vi "mainhex.vi"() -> ()   [LabVIEW 2018]
uses:
  <vilib>/Instr/_visa.llb/VISA Configure Serial Port (Instr).vi
panel:
  out "Log file path":path
  in  "Project Name":string="BDC_prototype"
  out "Bat current":dbl caption="Current Temperature\n(Celsius)"
  out "Bat current":cluster{dbl[], dbl[]}(graph)
  out "Bat Voltage":dbl caption="Current Temperature\n(Celsius)"
  out "Bat voltage":cluster{dbl[], dbl[]}(graph)
  out "Time":dbl caption="Current Temperature\n(Celsius)"
  out "String":string
  in  "stop":bool
  out "Bus Voltage":dbl caption="Current Temperature\n(Celsius)"
  out "Bus voltage":cluster{dbl[], dbl[]}(graph)
  in  "Port":refnum<visa-resource-name>="COM5"
  in  "Baud rate":u32=57600
  in  "Data bits (8)":u16=8 min=5 max=8 step=1
  in  "Stop bits (1)":u16(ring)=10 items=["1.0"=10, "1.5"=15, "2.0"=20]
  in  "Flow control (None)":u16(ring) items=["None", "XON/XOFF", "RTS/CTS", "XON/XOFF & RTS/CTS", "DTR/DSR", "XON/XOFF & DTR/DSR"]
  in  "Parity (None)":enum16{"None", "Odd", "Even", "Mark", "Space"}(ring)
  # "UART"
  # "FILES"
  # "ACTIONS"
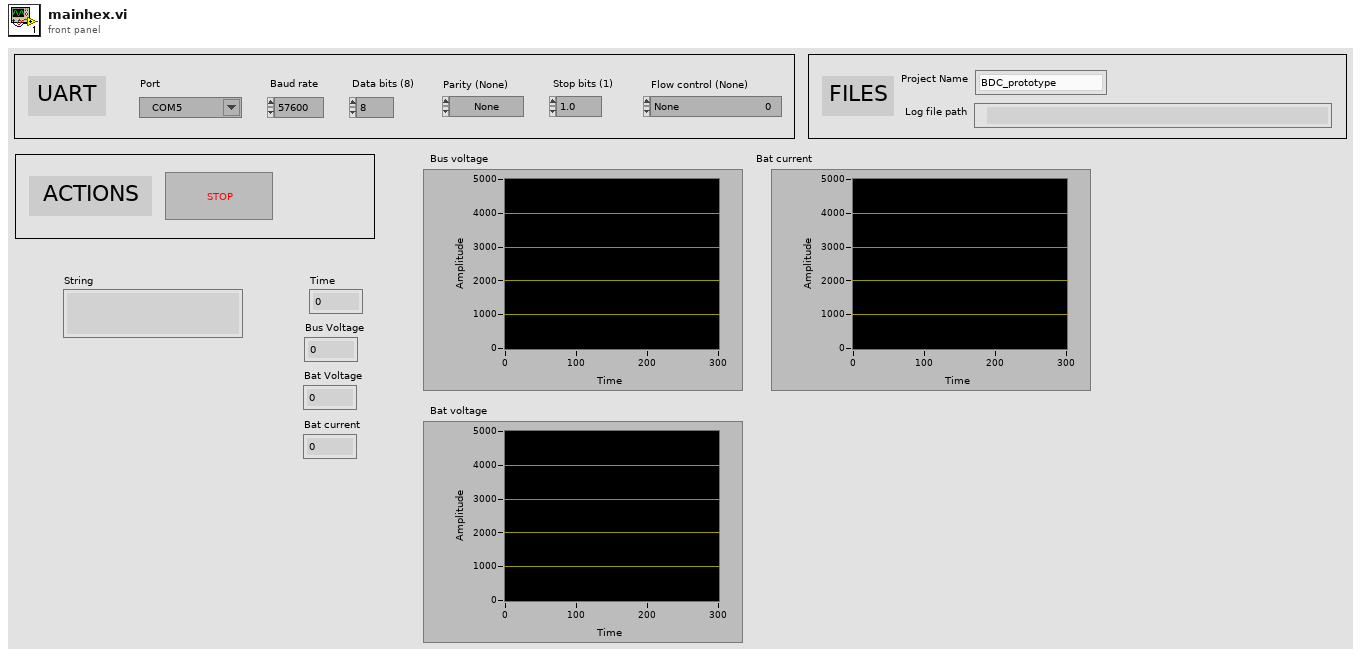
[diagram p1: front panel]
types:
  T1 = enum16{"open", "open or create", "create or replace", "create", "open (read only)"}
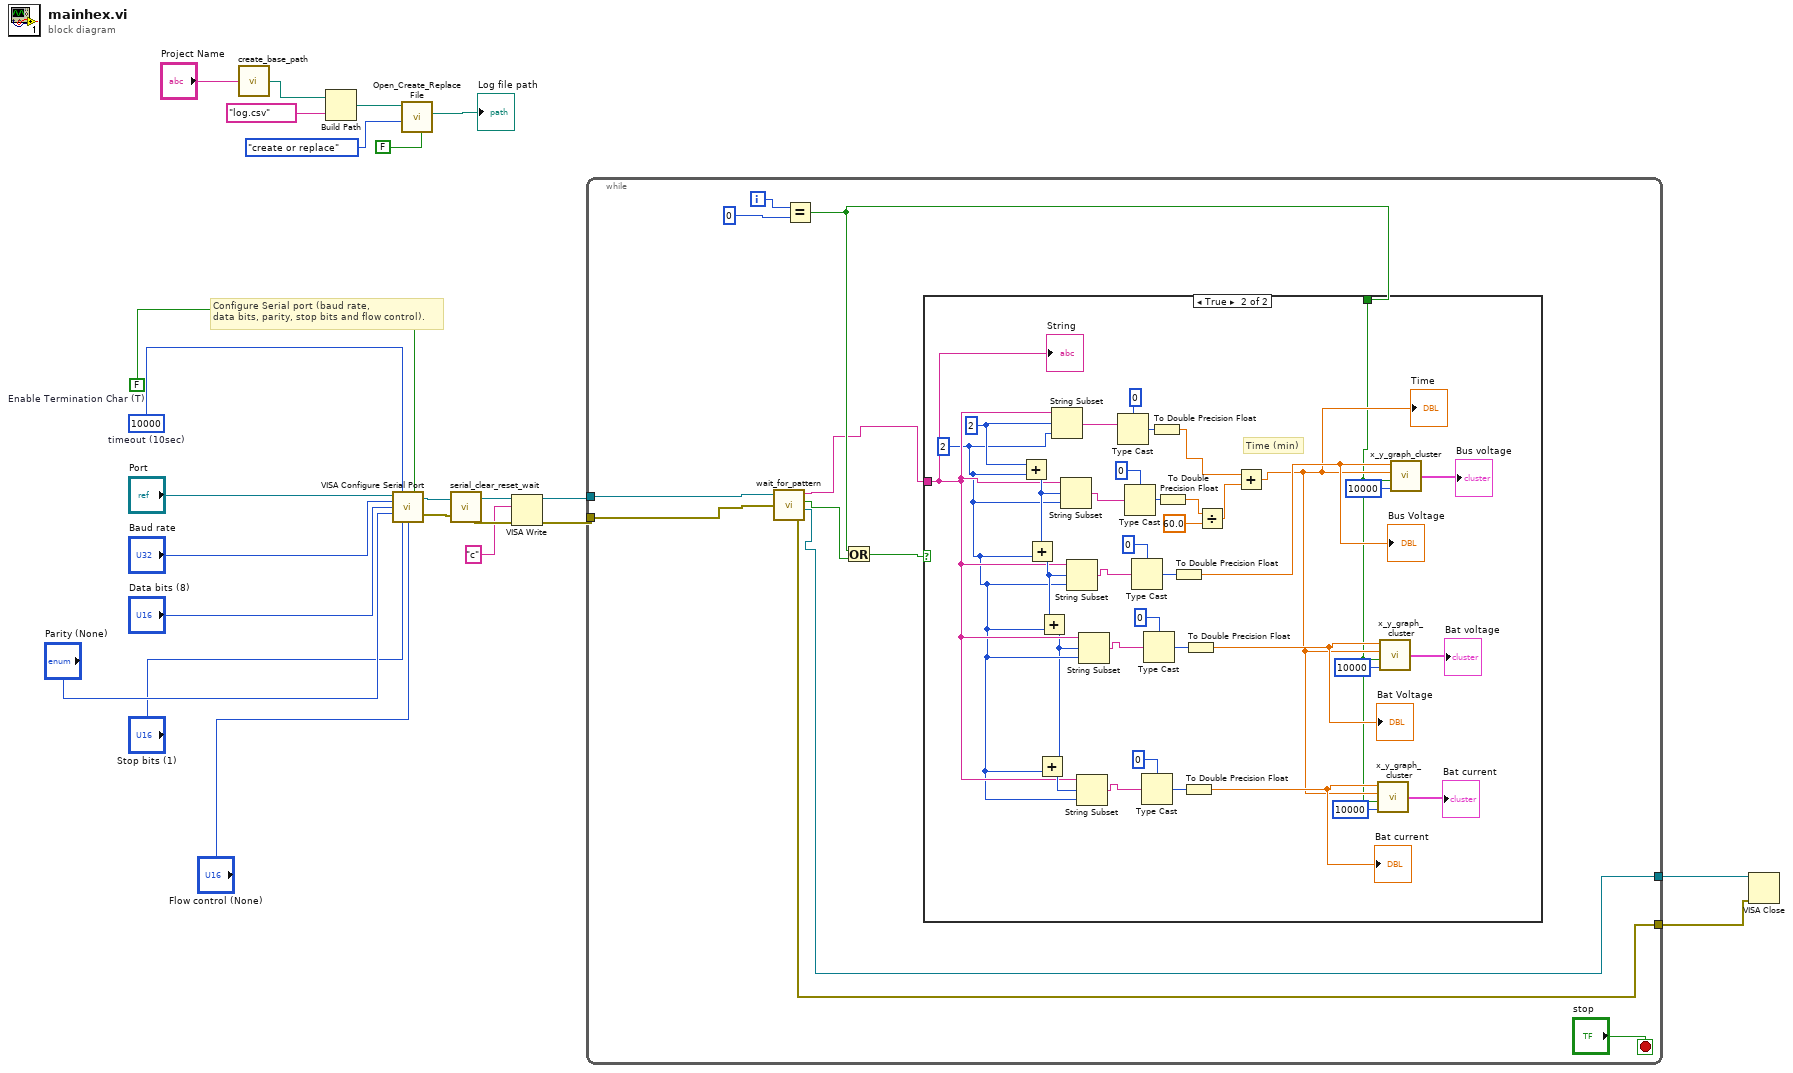
[diagram p0: block diagram]
diagram:
  w23 = FALSE  # Enable Termination Char (T)
  w24 = u32 10000  # timeout (10sec)
  # "Configure Serial port (baud rate,\ndata bits, parity, stop bits and flow control)."
  n1 = call "create_base_path.vi"("project name"="Project Name") -> ("base path"=w9:path)
  n2 = Build Path(base path=w9, name or relative path="log.csv") -> (appended path=w13:path)
  n3 = call-poly "VISA Configure Serial Port"("VISA resource name"="Port", "timeout (10sec)"=w24, "Enable Termination\nChar (T)"=w23, "baud rate (9600)"="Baud rate", "data bits (8)"="Data bits (8)", "parity (0:none)"="Parity (None)", "stop bits (10: 1 bit)"="Stop bits (1)", "flow control (0:none)"="Flow control (None)") -> ("VISA resource name out"=w21:refnum<visa-resource-name>, "error out"=w22:errorcluster)  [unwired: 6 in]
  n4 = call <vilib>:"Open_Create_Replace File.vi"("advisory dialog? (display:T)"=FALSE, "function (open:0)"=T1."create or replace", "file path"=w13) -> ("new file path"=→"Log file path":path)  [unwired: 5 in, 3 out]
  n5 = call "serial_clear_reset_wait.vi"("error in (no error)"=w22, "VISA Refnum in"=w21) -> ("error out"=w4:errorcluster, "VISA Refnum out"=w5:refnum<visa-resource-name>)
  n6 = VISA Write(VISA resource name=w5, write buffer="c", error in (no error)=w4) -> (VISA resource name out=w3:refnum<visa-resource-name>, error out=w2:errorcluster)  [unwired: 1 out]
  n7 = while {
    tunnel: w3 -> [w35]
    tunnel: w2 -> [w34]
    tunnel: [w28] -> w7
    tunnel: [w27] -> w6
    i -> [w29]
    stop <- "stop" stop-if-true
    n8 = call "wait_for_pattern.vi"("serial in"=w35, "error in (no error)"=w34) -> ("pattern string"=w25:string, "pattern detected"=w32:bool, "serial out"=w27:refnum<visa-resource-name>, "error out"=w28:errorcluster)  [unwired: 1 in]
    n9 = Equal?(x=w29, y=0) -> (x = y?=w30:bool)
    n10 = Or(x=w30, y=w32) -> (x .or. y?=w26:bool)
    n11 = case shown="True" w26 {
      tunnel: w25 -> [_ w40]
      tunnel: w30 -> [_ w36]
      frame False {
      }
      frame True {
        w39 = 2 ("length (rest)")
        w72 = 2 ("offset (0)")
        # "Time (min)"
        n12 = Add(x=w72, y=w39) -> (x+y=w69:i32)
        n13 = Add(x=w69, y=w39) -> (x+y=w51:i32)
        n14 = Add(x=w51, y=w39) -> (x+y=w38:i32)
        n15 = Add(x=w38, y=w39) -> (x+y=w47:i32)
        n16 = String Subset(string=w40, offset (0)=w72, length (rest)=w39) -> (substring=w63:string)
        n17 = String Subset(string=w40, offset (0)=w69, length (rest)=w39) -> (substring=w59:string)
        n18 = String Subset(string=w40, offset (0)=w51, length (rest)=w39) -> (substring=w67:string)
        n19 = String Subset(string=w40, offset (0)=w47, length (rest)=w39) -> (substring=w46:string)
        n20 = String Subset(string=w40, offset (0)=w38, length (rest)=w39) -> (substring=w54:string)
        n21 = Type Cast(type=u16 0 ("default (0 U32)"), x=w63) -> (*(type *) &x=w56:u16)
        n22 = Type Cast(type=u16 0 ("default (0 U32)"), x=w59) -> (*(type *) &x=w58:u16)
        n23 = Type Cast(type=u16 0 ("default (0 U32)"), x=w67) -> (*(type *) &x=w62:u16)
        n24 = Type Cast(type=u16 0 ("default (0 U32)"), x=w46) -> (*(type *) &x=w44:u16)
        n25 = Type Cast(type=u16 0 ("default (0 U32)"), x=w54) -> (*(type *) &x=w52:u16)
        n26 = To Double Precision Float(number=w56) -> (double precision float=w55:dbl)
        n27 = To Double Precision Float(number=w58) -> (double precision float=w57:dbl)
        n28 = To Double Precision Float(number=w62) -> (double precision float=w61:dbl)
        "Bus Voltage" <- w61
        n29 = To Double Precision Float(number=w44) -> (double precision float=w41:dbl)
        "Bat current" <- w41
        n30 = To Double Precision Float(number=w52) -> (double precision float=w48:dbl)
        "Bat Voltage" <- w48
        n31 = Divide(x=w57, y=60.0) -> (x/y=w70:dbl)
        n32 = Add(x=w55, y=w70) -> (x+y=w37:dbl)
        "Time" <- w37
        n33 = call "x_y_graph_cluster.vi"("Chart History (10,000)"=10000, "Clear Graph?"=w36, "X"=w37, "Y"=w41) -> ("Cluster"=→"Bat current":cluster{dbl[], dbl[]})
        n34 = call "x_y_graph_cluster.vi"("Chart History (10,000)"=10000, "Clear Graph?"=w36, "X"=w37, "Y"=w48) -> ("Cluster"=→"Bat voltage":cluster{dbl[], dbl[]})
        n35 = call "x_y_graph_cluster.vi"("Chart History (10,000)"=10000, "Clear Graph?"=w36, "X"=w37, "Y"=w61) -> ("Cluster"=→"Bus voltage":cluster{dbl[], dbl[]})
        "String" <- w40
      }
    }
  }
  n36 = VISA Close(VISA resource name=w6, error in (no error)=w7) -> ()  [unwired: 1 out]
